vi "Read password.vi"(8 "error in (no error)":errorcluster, 11 "protection settings in":refnum<class "protection settings.lvclass">) -> (0 "error out":errorcluster, 2 "password":string, 3 "protection settings out":refnum<class "protection settings.lvclass">)   [LabVIEW 2013, in "protection settings.lvclass"]
uses:
  protection settings.lvclass
  protection settings.lvclass/protection settings.ctl
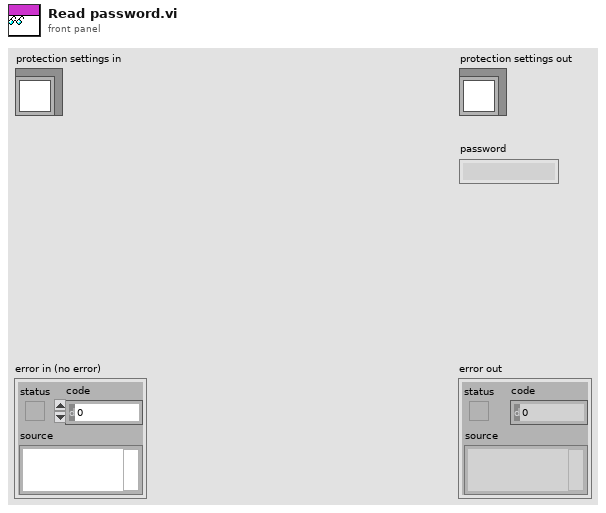
[diagram p1: front panel]
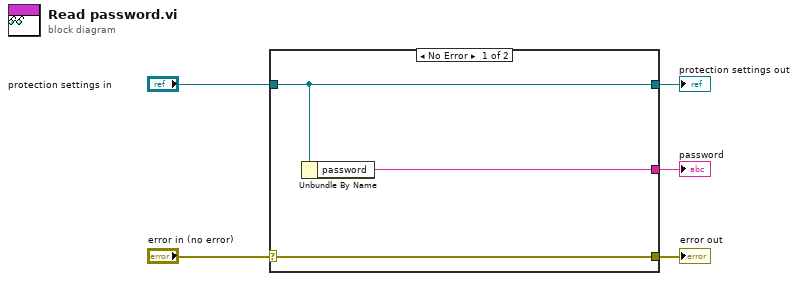
[diagram p0: block diagram]
diagram:
  n1 = case shown="No Error" "error in (no error)" {
    selector: "error in (no error)" -> [w8 w9]
    tunnel: [w8 w9] -> w4
    tunnel: [w7 w10] -> w2
    tunnel: "protection settings in" -> [w7 w10]
    tunnel: [w6 _] -> w1
    frame No Error {
      n2 = Unbundle By Name(w7) -> ("password"=w6:string)
    }
    frame Error {
    }
  }
  "error out" <- w4
  "protection settings out" <- w2
  "password" <- w1
